vi "Send command Set Pin.vi"(0 "NXP in":refnum<class "NXP.lvclass">, 1 "Puerto":string(combo), 2 "Pin":string(combo), 3 "Valor":string(combo), 5 "error in (no error)":errorcluster, 6 "Marca":string) -> (14 "NXP out":refnum<class "NXP.lvclass">, 16 "Command":string, 17 "Expected response":string, 19 "error out":errorcluster)   [LabVIEW 2020, in "NXP.lvclass"]
uses:
  NXP.lvclass
  NXP.lvclass/NXP.ctl
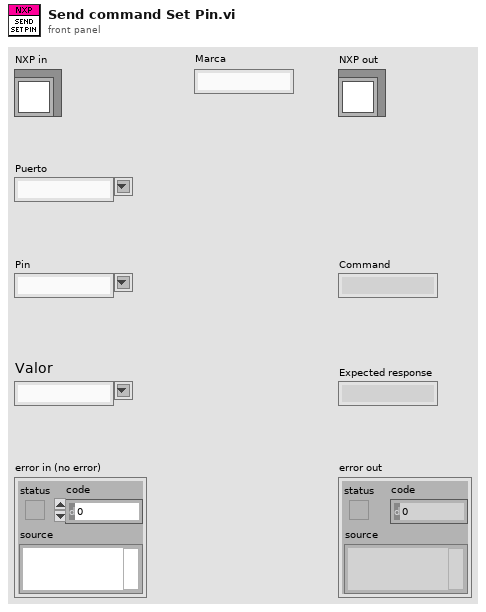
[diagram p1: front panel]
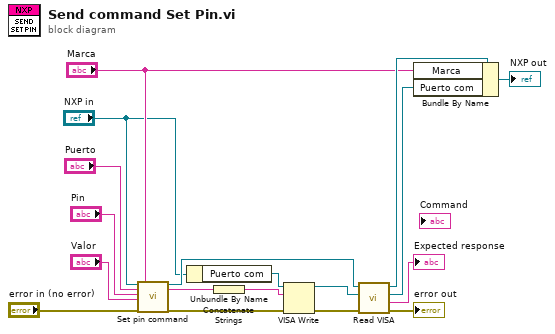
[diagram p0: block diagram]
diagram:
  n1 = call-dynamic "Set pin command.vi"("Serial Device in"="NXP in", "Puerto"="Puerto", "Pin"="Pin", "Valor"="Valor", "error in (no error)"="error in (no error)", "Marca"="Marca") -> ("Serial Device out"=w7:refnum<class "NXP.lvclass">, "Command"=w8:string, "error out"=w12:errorcluster)  [unwired: 10 in, 1 out]
  n2 = Unbundle By Name("NXP in") -> ("Puerto com"=w1:refnum<visa-resource-name>)
  n3 = Concatenate Strings(w8) -> (w9:string)
  n4 = VISA Write(VISA resource name=w1, write buffer=w9, error in (no error)=w12) -> (VISA resource name out=w14:refnum<visa-resource-name>, error out=w13:errorcluster)  [unwired: 1 out]
  n5 = call-dynamic "Read VISA.vi"("error in (no error)"=w13, "VISA Refnum in"=w14, "Serial Device in"=w7) -> ("error out"=→"error out":errorcluster, "Serial Response"=→"Expected response":string, "VISA resource name out"=w3:refnum<visa-resource-name>, "Serial Device out"=w6:refnum<class "NXP.lvclass">)  [unwired: 5 in]
  n6 = Bundle By Name(cluster=w6, "Marca"="Marca", "Puerto com"=w3) -> (→"NXP out":refnum<class "NXP.lvclass">)
